vi "Global M2.vi"() -> ()   [LabVIEW 2017]
panel:
  in  "Locked!":bool
  in  "Jump!":bool
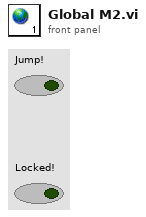
[diagram p1: front panel]
diagram:
